vi "操作日志.vi"(8 "error in (no error)":errorcluster, 10 "table":string="操作日志", 11 "日志信息":string) -> (0 "error out":errorcluster)   [LabVIEW 2016, in "斯坦道多参数.lvlib"]
uses:
  <vilib>/Utility/sysdir.llb/System Directory Type.ctl
  <vilib>/addons/database/Auxilliary.llb/DB Tools Transaction.ctl
  <vilib>/addons/database/Auxilliary.llb/DB Tools Isolation Level.ctl
  <vilib>/addons/database/Connection.llb/DB Tools Open Connec (String).vi
  <vilib>/addons/database/Connection.llb/Conn Transaction.vi
  <vilib>/addons/database/NI_Database_API.lvlib
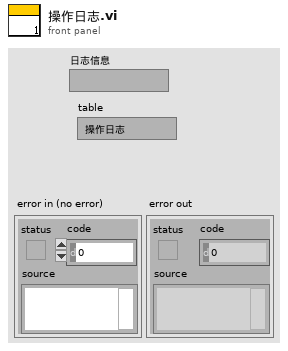
[diagram p1: front panel]
types:
  T1 = typedef "NI_Database_API.lvlib/DB Tools Isolation Level.ctl" = enum16{"chaos", "read uncommitted", "read committed", "repeatable read", "serializable"}
  T2 = typedef "NI_Database_API.lvlib/DB Tools Transaction.ctl" = enum16{"begin", "commit", "rollback"}
  T3 = cluster{"时间标识":timestamp, "设备":string, "日志信息":string, "流程参数":string}
  T4 = typedef "System Directory Type.ctl" = i32
  T5 = typedef "NI_Database_API.lvlib/Conn ObjectReference.ctl" = refnum<k1>
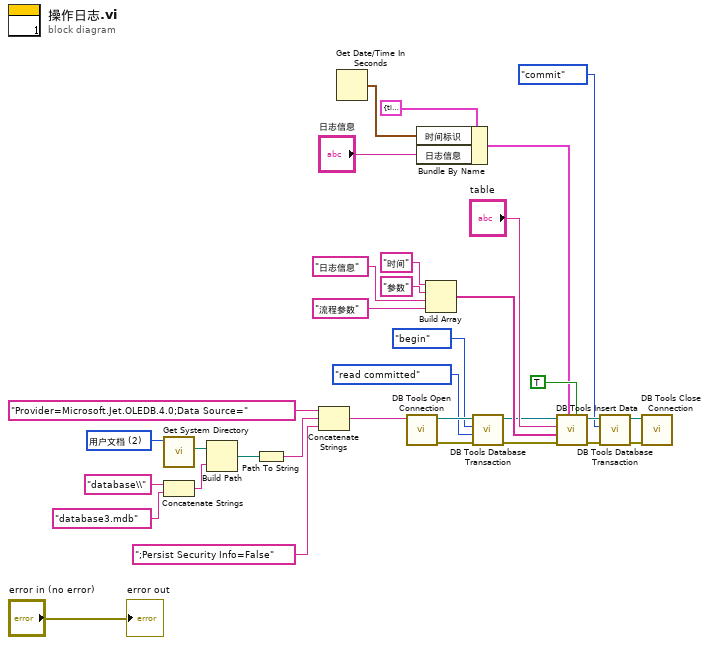
[diagram p0: block diagram]
diagram:
  w28 = T4 2 items=["用户目录"=0, "用户桌面"=1, "用户文档"=2, "用户应用程序数据"=3, "用户设置"=4, "用户临时目录"=5, "公共文档"=6, "公共应用程序数据"=7, "公共设置"=8, "公共缓存"=13, "系统核心库"=9, "系统安装库"=10, "应用程序文件"=11, "启动盘根目录"=12] ("system directory type")
  n1 = call <vilib>:"Get System Directory.vi"("system directory type"=w28) -> ("system directory"=w26:path)  [unwired: 10 in]
  n2 = Concatenate Strings("database\\" ("condition"), "database3.mdb" ("database")) -> (w20:string)
  n3 = Build Path(base path=w26, name or relative path=w20) -> (appended path=w25:path)
  n4 = Path To String(path=w25) -> (string=w24:string)
  n5 = Concatenate Strings("Provider=Microsoft.Jet.OLEDB.4.0;Data Source=" ("condition"), w24, ";Persist Security Info=False" ("condition")) -> (w22:string)
  n6 = Get Date/Time In Seconds() -> (seconds since 1Jan1904=w13:timestamp)
  n7 = call-poly <vilib>:"DB Tools Open Connection.vi"("connection information"=w22) -> ("error out"=w9:errorcluster, "connection reference"=w19:T5)  [unwired: 7 in]
  n8 = Bundle By Name(cluster=T3 {"时间标识"=timestamp(0 s since 1904-01-01), "设备"="多参数", "日志信息"="", "流程参数"=""} ("data in"), "时间标识"=w13, "日志信息"="日志信息") -> (w12:T3)
  n9 = Build Array("时间", "参数" ("元素"), "日志信息", "流程参数") -> (w16:string[])
  n10 = call-poly <vilib>:"DB Tools Database Transaction.vi"("error in (no error)"=w9, "isolation level (chaos)"=DB_Tools_Isolation_Level."read committed", "operation (begin)"=DB_Tools_Transaction."begin", "connection reference"=w19) -> ("error out"=w8:errorcluster, "connection reference out"=w10:T5)  [unwired: 2 in]
  n11 = call <vilib>:"DB Tools Insert Data.vi"("create table? (F)"=TRUE, "data"=w12, "error in (no error)"=w8, "columns"=w16, "table"="table", "connection reference"=w10) -> ("error out"=w5:errorcluster, "connection reference out"=w7:T5)  [unwired: 4 in]
  n12 = call-poly <vilib>:"DB Tools Database Transaction.vi"("error in (no error)"=w5, "operation (begin)"=DB_Tools_Transaction."commit", "connection reference"=w7) -> ("error out"=w4:errorcluster, "connection reference out"=w6:T5)  [unwired: 3 in]
  n13 = call <vilib>:"DB Tools Close Connection.vi"("error in (no error)"=w4, "connection reference"=w6) -> ()  [unwired: 5 in, 1 out]
  "error out" <- "error in (no error)"
